vi "Configure Marker.vi"(0 "VISA resource name":refnum<visa-resource-name>, 1 "Marker X Position (1E3)":dbl=1000.0 format="%^#_9g", 2 "Enable Coupling (Disable)":bool, 3 "Enable Reference Mode (Disable)":bool, 5 "Measurement Type (6: Phase Noise)":u16(ring)=6 items=["AM Noise"=1, "Baseband Noise"=2, "Freq/Power"=3, "Spectrum"=4, "Transient"=5, "Phase Noise"=6, "User"=7], 7 "Select Trace (1: 1)":u16(ring)=1 items=["1"=1, "2"=2, "3"=3, "4"=4, "5"=5, "6"=6, "7"=7, "8"=8], 9 "Select Marker (1: 1)":u16(ring)=1 items=["1"=1, "2"=2, "3"=3, "4"=4, "5"=5, "6"=6, "7"=7, "8"=8, "9"=9, "10"=10], 11 "error in (no error)":errorcluster, 12 "Enable Marker (Enable)":bool=TRUE, 13 "Tracking Mode (4: Off)":T1(ring)=enum."Off") -> (4 "VISA resource name out":refnum<visa-resource-name>, 15 "error out":errorcluster)   [LabVIEW 2011, in "Agilent E5052X.lvlib"]
doc: "Configures markers to be used in measurements. Use multiple instances of this VI to configure multiple markers. \n\n<b>Note: </b>\n\nThis VI does not configure the search properties of the markers. Use the \"Configure Marker Search\" VI for that kind of functionality."
uses:
  Agilent E5052X.lvlib
panel:
  # "Marker Settings"
  # "Marker Function Settings"
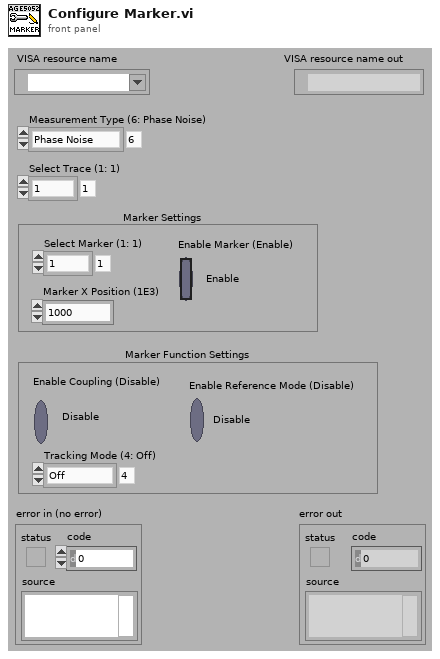
[diagram p1: front panel]
types:
  T1 = enum16{"Maximum", "Minimum", "Peak", "Target", "Off"}
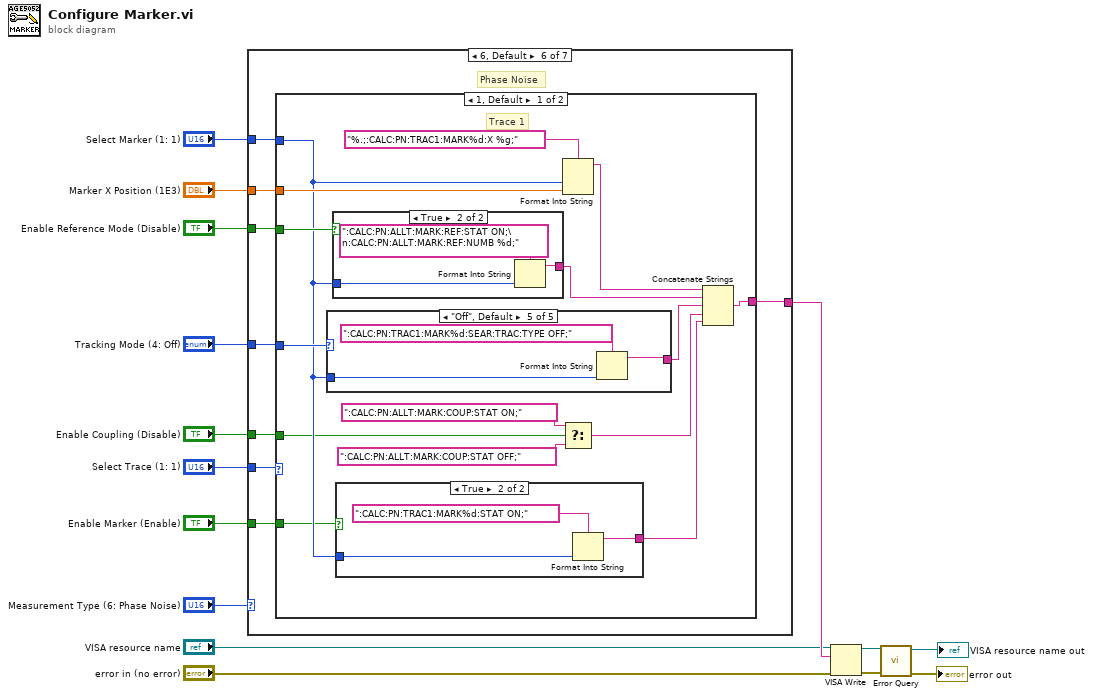
[diagram p0: block diagram]
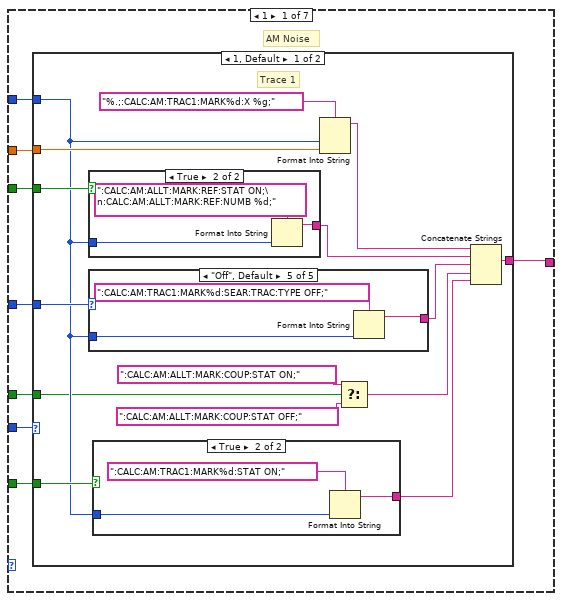
[diagram p2: hidden frame]
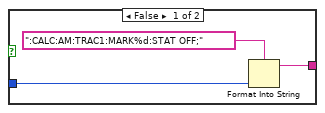
[diagram p3: hidden frame]
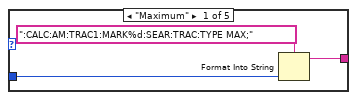
[diagram p4: hidden frame]
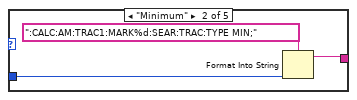
[diagram p5: hidden frame]
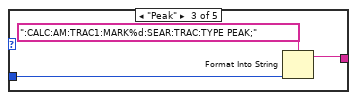
[diagram p6: hidden frame]
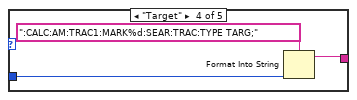
[diagram p7: hidden frame]
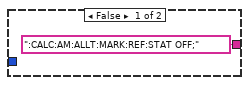
[diagram p8: hidden frame]
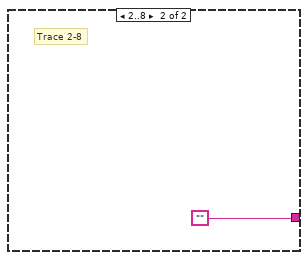
[diagram p9: hidden frame]
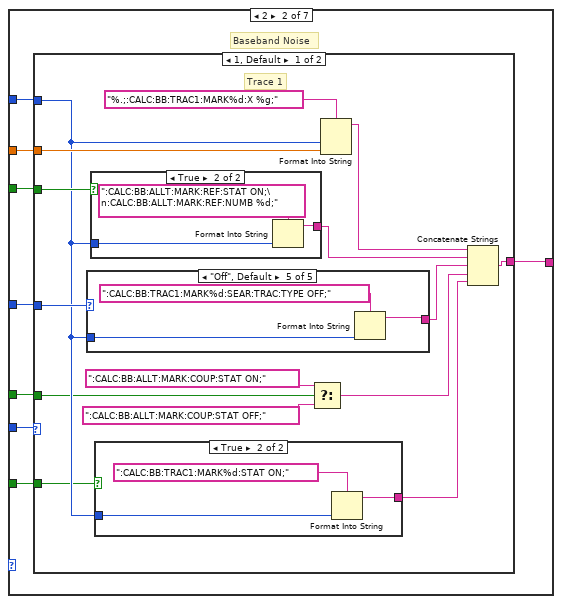
[diagram p10: hidden frame]
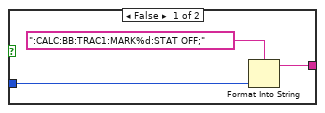
[diagram p11: hidden frame]
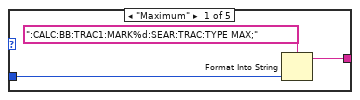
[diagram p12: hidden frame]
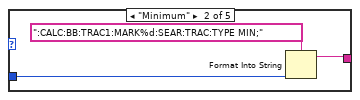
[diagram p13: hidden frame]
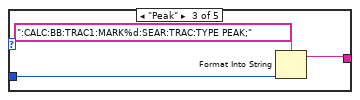
[diagram p14: hidden frame]
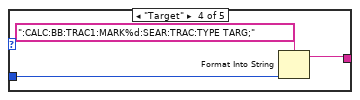
[diagram p15: hidden frame]
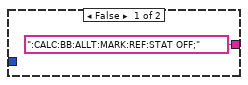
[diagram p16: hidden frame]
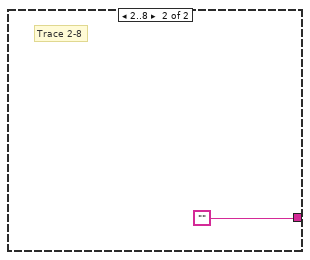
[diagram p17: hidden frame]
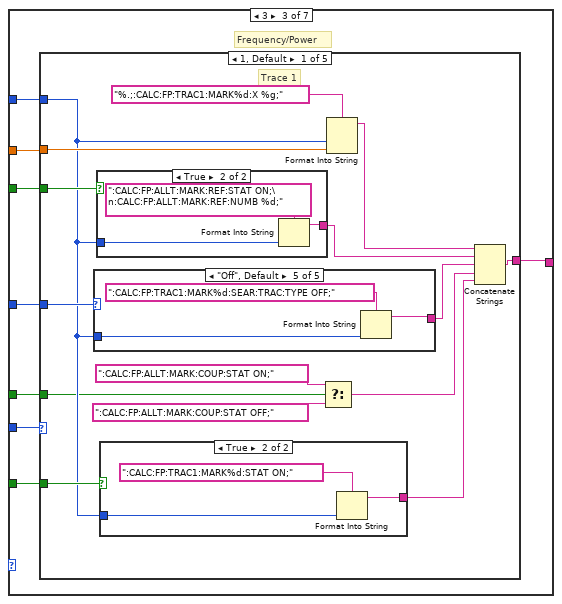
[diagram p18: hidden frame]
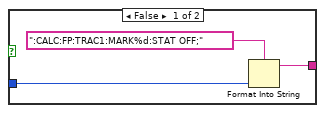
[diagram p19: hidden frame]
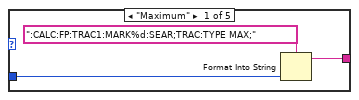
[diagram p20: hidden frame]
diagram:
  n1 = case shown="6, Default" "Measurement Type (6: Phase Noise)" {
    tunnel: "Enable Marker (Enable)" -> [w16 w65 w114 w283 w332 w501 w550]
    tunnel: "Select Trace (1: 1)" -> [w23 w67 w116 w285 w334 w503 w552]
    tunnel: "Select Marker (1: 1)" -> [w22 w72 w121 w290 w339 w508 w557]
    tunnel: "Enable Reference Mode (Disable)" -> [w21 w70 w119 w288 w337 w506 w555]
    tunnel: "Tracking Mode (4: Off)" -> [w20 w69 w118 w287 w336 w505 w554]
    tunnel: "Enable Coupling (Disable)" -> [w19 w68 w117 w286 w335 w504 w553]
    tunnel: "Marker X Position (1E3)" -> [w18 w71 w120 w289 w338 w507 w556]
    tunnel: [w17 w66 w115 w284 w333 w502 w551] -> w4
    frame 1 {
      # "AM Noise"
      n2 = case shown="1, Default" w23 {
        tunnel: w22 -> [w29 _]
        tunnel: w21 -> [w37 _]
        tunnel: w20 -> [w36 _]
        tunnel: w19 -> [w25 _]
        tunnel: w18 -> [w35 _]
        tunnel: [w31 ""] -> w17
        tunnel: w16 -> [w30 _]
        frame 1, Default {
          # "Trace 1"
          n3 = case shown="True" w37 {
            tunnel: w29 -> [_ w63]
            tunnel: [":CALC:AM:ALLT:MARK:REF:STAT OFF;" w61] -> w33
            frame False {
            }
            frame True {
              n4 = Format Into String(format string=":CALC:AM:ALLT:MARK:REF:STAT ON;\n:CALC:AM:ALLT:MARK:REF:NUMB %d;", w63) -> (resulting string=w61:string)  [unwired: 2 in, 1 out]
            }
          }
          n5 = case shown="\"Off\", Default" w36 {
            tunnel: w29 -> [w47 w49 w51 w54 w57]
            tunnel: [w45 w48 w52 w55 w58] -> w32
            frame "Maximum" {
              n6 = Format Into String(format string=":CALC:AM:TRAC1:MARK%d:SEAR:TRAC:TYPE MAX;", w47) -> (resulting string=w45:string)  [unwired: 2 in, 1 out]
            }
            frame "Minimum" {
              n7 = Format Into String(format string=":CALC:AM:TRAC1:MARK%d:SEAR:TRAC:TYPE MIN;", w49) -> (resulting string=w48:string)  [unwired: 2 in, 1 out]
            }
            frame "Peak" {
              n8 = Format Into String(format string=":CALC:AM:TRAC1:MARK%d:SEAR:TRAC:TYPE PEAK;", w51) -> (resulting string=w52:string)  [unwired: 2 in, 1 out]
            }
            frame "Target" {
              n9 = Format Into String(format string=":CALC:AM:TRAC1:MARK%d:SEAR:TRAC:TYPE TARG;", w54) -> (resulting string=w55:string)  [unwired: 2 in, 1 out]
            }
            frame "Off", Default {
              n10 = Format Into String(format string=":CALC:AM:TRAC1:MARK%d:SEAR:TRAC:TYPE OFF;", w57) -> (resulting string=w58:string)  [unwired: 2 in, 1 out]
            }
          }
          n11 = case shown="True" w30 {
            tunnel: w29 -> [w40 w43]
            tunnel: [w39 w42] -> w28
            frame False {
              n12 = Format Into String(format string=":CALC:AM:TRAC1:MARK%d:STAT OFF;", w40) -> (resulting string=w39:string)  [unwired: 2 in, 1 out]
            }
            frame True {
              n13 = Format Into String(format string=":CALC:AM:TRAC1:MARK%d:STAT ON;", w43) -> (resulting string=w42:string)  [unwired: 2 in, 1 out]
            }
          }
          n14 = Format Into String(format string="%.;:CALC:AM:TRAC1:MARK%d:X %g;", w29, w35) -> (resulting string=w34:string)  [unwired: 2 in, 1 out]
          n15 = Select(t=":CALC:AM:ALLT:MARK:COUP:STAT ON;", s=w25, f=":CALC:AM:ALLT:MARK:COUP:STAT OFF;") -> (s? t:f=w24:string)
          n16 = Concatenate Strings(w34, w33, w32, w24, w28) -> (w31:string)
        }
        frame 2..8 {
          # "Trace 2-8"
        }
      }
    }
    frame 2 {
      # "Baseband Noise"
      n17 = case shown="1, Default" w67 {
        tunnel: w72 -> [w79 _]
        tunnel: w70 -> [w86 _]
        tunnel: w69 -> [w85 _]
        tunnel: w68 -> [w74 _]
        tunnel: w71 -> [w84 _]
        tunnel: [w80 ""] -> w66
        tunnel: w65 -> [w78 _]
        frame 1, Default {
          # "Trace 1"
          n18 = case shown="\"Off\", Default" w85 {
            tunnel: w79 -> [w96 w98 w100 w103 w106]
            tunnel: [w94 w97 w101 w104 w107] -> w81
            frame "Maximum" {
              n19 = Format Into String(format string=":CALC:BB:TRAC1:MARK%d:SEAR:TRAC:TYPE MAX;", w96) -> (resulting string=w94:string)  [unwired: 2 in, 1 out]
            }
            frame "Minimum" {
              n20 = Format Into String(format string=":CALC:BB:TRAC1:MARK%d:SEAR:TRAC:TYPE MIN;", w98) -> (resulting string=w97:string)  [unwired: 2 in, 1 out]
            }
            frame "Peak" {
              n21 = Format Into String(format string=":CALC:BB:TRAC1:MARK%d:SEAR:TRAC:TYPE PEAK;", w100) -> (resulting string=w101:string)  [unwired: 2 in, 1 out]
            }
            frame "Target" {
              n22 = Format Into String(format string=":CALC:BB:TRAC1:MARK%d:SEAR:TRAC:TYPE TARG;", w103) -> (resulting string=w104:string)  [unwired: 2 in, 1 out]
            }
            frame "Off", Default {
              n23 = Format Into String(format string=":CALC:BB:TRAC1:MARK%d:SEAR:TRAC:TYPE OFF;", w106) -> (resulting string=w107:string)  [unwired: 2 in, 1 out]
            }
          }
          n24 = case shown="True" w86 {
            tunnel: w79 -> [_ w112]
            tunnel: [":CALC:BB:ALLT:MARK:REF:STAT OFF;" w110] -> w82
            frame False {
            }
            frame True {
              n25 = Format Into String(format string=":CALC:BB:ALLT:MARK:REF:STAT ON;\n:CALC:BB:ALLT:MARK:REF:NUMB %d;", w112) -> (resulting string=w110:string)  [unwired: 2 in, 1 out]
            }
          }
          n26 = case shown="True" w78 {
            tunnel: w79 -> [w89 w92]
            tunnel: [w88 w91] -> w77
            frame False {
              n27 = Format Into String(format string=":CALC:BB:TRAC1:MARK%d:STAT OFF;", w89) -> (resulting string=w88:string)  [unwired: 2 in, 1 out]
            }
            frame True {
              n28 = Format Into String(format string=":CALC:BB:TRAC1:MARK%d:STAT ON;", w92) -> (resulting string=w91:string)  [unwired: 2 in, 1 out]
            }
          }
          n29 = Select(t=":CALC:BB:ALLT:MARK:COUP:STAT ON;", s=w74, f=":CALC:BB:ALLT:MARK:COUP:STAT OFF;") -> (s? t:f=w73:string)
          n30 = Format Into String(format string="%.;:CALC:BB:TRAC1:MARK%d:X %g;", w79, w84) -> (resulting string=w83:string)  [unwired: 2 in, 1 out]
          n31 = Concatenate Strings(w83, w82, w81, w73, w77) -> (w80:string)
        }
        frame 2..8 {
          # "Trace 2-8"
        }
      }
    }
    frame 3 {
      # "Frequency/Power"
      n32 = case shown="1, Default" w116 {
        tunnel: w121 -> [w127 w168 w207 w248 _]
        tunnel: w119 -> [w135 w171 w211 w251 _]
        tunnel: w118 -> [w134 w170 w210 w250 _]
        tunnel: w117 -> [w123 w163 w203 w243 _]
        tunnel: w120 -> [w133 w172 w212 w252 _]
        tunnel: [w129 w169 w209 w249 ""] -> w115
        tunnel: w114 -> [w128 w167 w208 w247 _]
        frame 1, Default {
          # "Trace 1"
          n33 = case shown="\"Off\", Default" w134 {
            tunnel: w127 -> [w145 w147 w149 w152 w155]
            tunnel: [w143 w146 w150 w153 w156] -> w130
            frame "Maximum" {
              n34 = Format Into String(format string=":CALC:FP:TRAC1:MARK%d:SEAR;TRAC:TYPE MAX;", w145) -> (resulting string=w143:string)  [unwired: 2 in, 1 out]
            }
            frame "Minimum" {
              n35 = Format Into String(format string=":CALC:FP:TRAC1:MARK%d:SEAR;TRAC:TYPE MIN;", w147) -> (resulting string=w146:string)  [unwired: 2 in, 1 out]
            }
            frame "Peak" {
              n36 = Format Into String(format string=":CALC:FP:TRAC1:MARK%d:SEAR;TRAC:TYPE PEAK;", w149) -> (resulting string=w150:string)  [unwired: 2 in, 1 out]
            }
            frame "Target" {
              n37 = Format Into String(format string=":CALC:FP:TRAC1:MARK%d:SEAR;TRAC:TYPE TARG;", w152) -> (resulting string=w153:string)  [unwired: 2 in, 1 out]
            }
            frame "Off", Default {
              n38 = Format Into String(format string=":CALC:FP:TRAC1:MARK%d:SEAR:TRAC:TYPE OFF;", w155) -> (resulting string=w156:string)  [unwired: 2 in, 1 out]
            }
          }
          n39 = case shown="True" w135 {
            tunnel: w127 -> [_ w161]
            tunnel: [":CALC:FP:ALLT:MARK:REF:STAT OFF;" w159] -> w131
            frame False {
            }
            frame True {
              n40 = Format Into String(format string=":CALC:FP:ALLT:MARK:REF:STAT ON;\n:CALC:FP:ALLT:MARK:REF:NUMB %d;", w161) -> (resulting string=w159:string)  [unwired: 2 in, 1 out]
            }
          }
          n41 = case shown="True" w128 {
            tunnel: w127 -> [w138 w141]
            tunnel: [w137 w140] -> w126
            frame False {
              n42 = Format Into String(format string=":CALC:FP:TRAC1:MARK%d:STAT OFF;", w138) -> (resulting string=w137:string)  [unwired: 2 in, 1 out]
            }
            frame True {
              n43 = Format Into String(format string=":CALC:FP:TRAC1:MARK%d:STAT ON;", w141) -> (resulting string=w140:string)  [unwired: 2 in, 1 out]
            }
          }
          n44 = Select(t=":CALC:FP:ALLT:MARK:COUP:STAT ON;", s=w123, f=":CALC:FP:ALLT:MARK:COUP:STAT OFF;") -> (s? t:f=w122:string)
          n45 = Format Into String(format string="%.;:CALC:FP:TRAC1:MARK%d:X %g;", w127, w133) -> (resulting string=w132:string)  [unwired: 2 in, 1 out]
          n46 = Concatenate Strings(w132, w131, w130, w122, w126) -> (w129:string)
        }
        frame 2 {
          # "Trace 2"
          n47 = case shown="\"Off\", Default" w170 {
            tunnel: w168 -> [w185 w187 w189 w192 w195]
            tunnel: [w183 w186 w190 w193 w196] -> w173
            frame "Maximum" {
              n48 = Format Into String(format string=":CALC:FP:TRAC2:MARK%d:SEAR:TRAC:TYPE MAX;", w185) -> (resulting string=w183:string)  [unwired: 2 in, 1 out]
            }
            frame "Minimum" {
              n49 = Format Into String(format string=":CALC:FP:TRAC2:MARK%d:SEAR:TRAC:TYPE MIN;", w187) -> (resulting string=w186:string)  [unwired: 2 in, 1 out]
            }
            frame "Peak" {
              n50 = Format Into String(format string=":CALC:FP:TRAC2:MARK%d:SEAR:TRAC:TYPE PEAK;", w189) -> (resulting string=w190:string)  [unwired: 2 in, 1 out]
            }
            frame "Target" {
              n51 = Format Into String(format string=":CALC:FP:TRAC2:MARK%d:SEAR:TRAC:TYPE TARG;", w192) -> (resulting string=w193:string)  [unwired: 2 in, 1 out]
            }
            frame "Off", Default {
              n52 = Format Into String(format string=":CALC:FP:TRAC2:MARK%d:SEAR:TRAC:TYPE OFF;", w195) -> (resulting string=w196:string)  [unwired: 2 in, 1 out]
            }
          }
          n53 = case shown="True" w171 {
            tunnel: w168 -> [_ w201]
            tunnel: [":CALC:FP:ALLT:MARK:REF:STAT OFF;" w199] -> w174
            frame False {
            }
            frame True {
              n54 = Format Into String(format string=":CALC:FP:ALLT:MARK:REF:STAT ON;\n:CALC:FP:ALLT:MARK:REF:NUMB %d;", w201) -> (resulting string=w199:string)  [unwired: 2 in, 1 out]
            }
          }
          n55 = case shown="True" w167 {
            tunnel: w168 -> [w178 w181]
            tunnel: [w177 w180] -> w166
            frame False {
              n56 = Format Into String(format string=":CALC:FP:TRAC2:MARK%d:STAT OFF;", w178) -> (resulting string=w177:string)  [unwired: 2 in, 1 out]
            }
            frame True {
              n57 = Format Into String(format string=":CALC:FP:TRAC2:MARK%d:STAT ON;", w181) -> (resulting string=w180:string)  [unwired: 2 in, 1 out]
            }
          }
          n58 = Select(t=":CALC:FP:ALLT:MARK:COUP:STAT ON;", s=w163, f=":CALC:FP:ALLT:MARK:COUP:STAT OFF;") -> (s? t:f=w162:string)
          n59 = Format Into String(format string="%.;:CALC:FP:TRAC2:MARK%d:X %g;", w168, w172) -> (resulting string=w175:string)  [unwired: 2 in, 1 out]
          n60 = Concatenate Strings(w175, w174, w173, w162, w166) -> (w169:string)
        }
        frame 3 {
          # "Trace 3"
          n61 = case shown="\"Off\", Default" w210 {
            tunnel: w207 -> [w225 w227 w229 w232 w235]
            tunnel: [w223 w226 w230 w233 w236] -> w213
            frame "Maximum" {
              n62 = Format Into String(format string=":CALC:FP:TRAC3:MARK%d:SEAR:TRAC:TYPE MAX;", w225) -> (resulting string=w223:string)  [unwired: 2 in, 1 out]
            }
            frame "Minimum" {
              n63 = Format Into String(format string=":CALC:FP:TRAC3:MARK%d:SEAR:TRAC:TYPE MIN;", w227) -> (resulting string=w226:string)  [unwired: 2 in, 1 out]
            }
            frame "Peak" {
              n64 = Format Into String(format string=":CALC:FP:TRAC3:MARK%d:SEAR:TRAC:TYPE PEAK;", w229) -> (resulting string=w230:string)  [unwired: 2 in, 1 out]
            }
            frame "Target" {
              n65 = Format Into String(format string=":CALC:FP:TRAC3:MARK%d:SEAR:TRAC:TYPE TARG;", w232) -> (resulting string=w233:string)  [unwired: 2 in, 1 out]
            }
            frame "Off", Default {
              n66 = Format Into String(format string=":CALC:FP:TRAC3:MARK%d:SEAR:TRAC:TYPE OFF;", w235) -> (resulting string=w236:string)  [unwired: 2 in, 1 out]
            }
          }
          n67 = case shown="True" w211 {
            tunnel: w207 -> [_ w241]
            tunnel: [":CALC:FP:ALLT:MARK:REF:STAT OFF;" w239] -> w214
            frame False {
            }
            frame True {
              n68 = Format Into String(format string=":CALC:FP:ALLT:MARK:REF:STAT ON;\n:CALC:FP:ALLT:MARK:REF:NUMB %d;", w241) -> (resulting string=w239:string)  [unwired: 2 in, 1 out]
            }
          }
          n69 = case shown="True" w208 {
            tunnel: w207 -> [w218 w221]
            tunnel: [w217 w220] -> w206
            frame False {
              n70 = Format Into String(format string=":CALC:FP:TRAC3:MARK%d:STAT OFF;", w218) -> (resulting string=w217:string)  [unwired: 2 in, 1 out]
            }
            frame True {
              n71 = Format Into String(format string=":CALC:FP:TRAC3:MARK%d:STAT ON;", w221) -> (resulting string=w220:string)  [unwired: 2 in, 1 out]
            }
          }
          n72 = Format Into String(format string="%.;:CALC:FP:TRAC3:MARK%d:X %g;", w207, w212) -> (resulting string=w215:string)  [unwired: 2 in, 1 out]
          n73 = Select(t=":CALC:FP:ALLT:MARK:COUP:STAT ON;", s=w203, f=":CALC:FP:ALLT:MARK:COUP:STAT OFF;") -> (s? t:f=w202:string)
          n74 = Concatenate Strings(w215, w214, w213, w202, w206) -> (w209:string)
        }
        frame 4 {
          # "Trace 4"
          n75 = case shown="\"Off\", Default" w250 {
            tunnel: w248 -> [w265 w267 w269 w272 w275]
            tunnel: [w263 w266 w270 w273 w276] -> w253
            frame "Maximum" {
              n76 = Format Into String(format string=":CALC:FP:TRAC4:MARK%d:SEAR:TRAC:TYPE MAX;", w265) -> (resulting string=w263:string)  [unwired: 2 in, 1 out]
            }
            frame "Minimum" {
              n77 = Format Into String(format string=":CALC:FP:TRAC4:MARK%d:SEAR:TRAC:TYPE MIN;", w267) -> (resulting string=w266:string)  [unwired: 2 in, 1 out]
            }
            frame "Peak" {
              n78 = Format Into String(format string=":CALC:FP:TRAC4:MARK%d:SEAR:TRAC:TYPE PEAK;", w269) -> (resulting string=w270:string)  [unwired: 2 in, 1 out]
            }
            frame "Target" {
              n79 = Format Into String(format string=":CALC:FP:TRAC4:MARK%d:SEAR:TRAC:TYPE TARG;", w272) -> (resulting string=w273:string)  [unwired: 2 in, 1 out]
            }
            frame "Off", Default {
              n80 = Format Into String(format string=":CALC:FP:TRAC4:MARK%d:SEAR:TRAC:TYPE OFF;", w275) -> (resulting string=w276:string)  [unwired: 2 in, 1 out]
            }
          }
          n81 = case shown="True" w251 {
            tunnel: w248 -> [_ w281]
            tunnel: [":CALC:FP:ALLT:MARK:REF:STAT OFF;" w279] -> w254
            frame False {
            }
            frame True {
              n82 = Format Into String(format string=":CALC:FP:ALLT:MARK:REF:STAT ON;\n:CALC:FP:ALLT:MARK:REF:NUMB %d;", w281) -> (resulting string=w279:string)  [unwired: 2 in, 1 out]
            }
          }
          n83 = case shown="True" w247 {
            tunnel: w248 -> [w258 w261]
            tunnel: [w257 w260] -> w246
            frame False {
              n84 = Format Into String(format string=":CALC:FP:TRAC4:MARK%d:STAT OFF;", w258) -> (resulting string=w257:string)  [unwired: 2 in, 1 out]
            }
            frame True {
              n85 = Format Into String(format string=":CALC:FP:TRAC4:MARK%d:STAT ON;", w261) -> (resulting string=w260:string)  [unwired: 2 in, 1 out]
            }
          }
          n86 = Format Into String(format string="%.;:CALC:FP:TRAC4:MARK%d:X %g;", w248, w252) -> (resulting string=w255:string)  [unwired: 2 in, 1 out]
          n87 = Select(t=":CALC:FP:ALLT:MARK:COUP:STAT ON;", s=w243, f=":CALC:FP:ALLT:MARK:COUP:STAT OFF;") -> (s? t:f=w242:string)
          n88 = Concatenate Strings(w255, w254, w253, w242, w246) -> (w249:string)
        }
        frame 5..8 {
          # "Trace 5-8"
        }
      }
    }
    frame 4 {
      # "Spectrum"
      n89 = case shown="1, Default" w285 {
        tunnel: w290 -> [w295 _]
        tunnel: w288 -> [w304 _]
        tunnel: w287 -> [w303 _]
        tunnel: w286 -> [w292 _]
        tunnel: w289 -> [w302 _]
        tunnel: [w298 ""] -> w284
        tunnel: w283 -> [w297 _]
        frame 1, Default {
          # "Trace 1"
          n90 = case shown="\"Off\", Default" w303 {
            tunnel: w295 -> [w314 w316 w318 w321 w324]
            tunnel: [w312 w315 w319 w322 w325] -> w299
            frame "Maximum" {
              n91 = Format Into String(format string=":CALC:SP:TRAC1:MARK%d:SEAR:TRAC:TYPE MAX;", w314) -> (resulting string=w312:string)  [unwired: 2 in, 1 out]
            }
            frame "Minimum" {
              n92 = Format Into String(format string=":CALC:SP:TRAC1:MARK%d:SEAR:TRAC:TYPE MIN;", w316) -> (resulting string=w315:string)  [unwired: 2 in, 1 out]
            }
            frame "Peak" {
              n93 = Format Into String(format string=":CALC:SP:TRAC1:MARK%d:SEAR:TRAC:TYPE PEAK;", w318) -> (resulting string=w319:string)  [unwired: 2 in, 1 out]
            }
            frame "Target" {
              n94 = Format Into String(format string=":CALC:SP:TRAC1:MARK%d:SEAR:TRAC:TYPE TARG;", w321) -> (resulting string=w322:string)  [unwired: 2 in, 1 out]
            }
            frame "Off", Default {
              n95 = Format Into String(format string=":CALC:SP:TRAC1:MARK%d:SEAR:TRAC:TYPE OFF;", w324) -> (resulting string=w325:string)  [unwired: 2 in, 1 out]
            }
          }
          n96 = case shown="True" w304 {
            tunnel: w295 -> [_ w330]
            tunnel: [":CALC:SP:ALLT:MARK:REF:STAT OFF;" w328] -> w300
            frame False {
            }
            frame True {
              n97 = Format Into String(format string=":CALC:SP:ALLT:MARK:REF:STAT ON;\n:CALC:SP:ALLT:MARK:REF:NUMB %d;", w330) -> (resulting string=w328:string)  [unwired: 2 in, 1 out]
            }
          }
          n98 = case shown="True" w297 {
            tunnel: w295 -> [w307 w310]
            tunnel: [w306 w309] -> w296
            frame False {
              n99 = Format Into String(format string=":CALC:SP:TRAC1:MARK%d:STAT OFF;", w307) -> (resulting string=w306:string)  [unwired: 2 in, 1 out]
            }
            frame True {
              n100 = Format Into String(format string=":CALC:SP:TRAC1:MARK%d:STAT ON;", w310) -> (resulting string=w309:string)  [unwired: 2 in, 1 out]
            }
          }
          n101 = Format Into String(format string="%.;:CALC:SP:TRAC1:MARK%d:X %g;", w295, w302) -> (resulting string=w301:string)  [unwired: 2 in, 1 out]
          n102 = Select(t=":CALC:SP:ALLT:MARK:COUP:STAT ON;", s=w292, f=":CALC:SP:ALLT:MARK:COUP:STAT OFF;") -> (s? t:f=w291:string)
          n103 = Concatenate Strings(w301, w300, w299, w291, w296) -> (w298:string)
        }
        frame 2..8 {
          # "Trace 2-8"
        }
      }
    }
    frame 5 {
      # "Transient"
      n104 = case shown="1, Default" w334 {
        tunnel: w339 -> [w344 w385 w425 w465 _]
        tunnel: w337 -> [w353 w389 w429 w469 _]
        tunnel: w336 -> [w352 w388 w428 w468 _]
        tunnel: w335 -> [w341 w381 w421 w461 _]
        tunnel: w338 -> [w351 w390 w430 w470 _]
        tunnel: [w347 w387 w427 w467 ""] -> w333
        tunnel: w332 -> [w345 w386 w426 w466 _]
        frame 1, Default {
          # "Trace 1"
          n105 = case shown="\"Off\", Default" w352 {
            tunnel: w344 -> [w363 w365 w367 w370 w373]
            tunnel: [w361 w364 w368 w371 w374] -> w348
            frame "Maximum" {
              n106 = Format Into String(format string=":CALC:TR:TRAC1:MARK%d:SEAR:TRAC:TYPE MAX;", w363) -> (resulting string=w361:string)  [unwired: 2 in, 1 out]
            }
            frame "Minimum" {
              n107 = Format Into String(format string=":CALC:TR:TRAC1:MARK%d:SEAR:TRAC:TYPE MIN;", w365) -> (resulting string=w364:string)  [unwired: 2 in, 1 out]
            }
            frame "Peak" {
              n108 = Format Into String(format string=":CALC:TR:TRAC1:MARK%d:SEAR:TRAC:TYPE PEAK;", w367) -> (resulting string=w368:string)  [unwired: 2 in, 1 out]
            }
            frame "Target" {
              n109 = Format Into String(format string=":CALC:TR:TRAC1:MARK%d:SEAR:TRAC:TYPE TARG;", w370) -> (resulting string=w371:string)  [unwired: 2 in, 1 out]
            }
            frame "Off", Default {
              n110 = Format Into String(format string=":CALC:TR:TRAC1:MARK%d:SEAR:TRAC:TYPE OFF;", w373) -> (resulting string=w374:string)  [unwired: 2 in, 1 out]
            }
          }
          n111 = case shown="True" w353 {
            tunnel: w344 -> [_ w379]
            tunnel: [":CALC:TR:ALLT:MARK:REF:STAT OFF;" w377] -> w349
            frame False {
            }
            frame True {
              n112 = Format Into String(format string=":CALC:TR:ALLT:MARK:REF:STAT ON;\n:CALC:TR:ALLT:MARK:REF:NUMB %d;", w379) -> (resulting string=w377:string)  [unwired: 2 in, 1 out]
            }
          }
          n113 = case shown="True" w345 {
            tunnel: w344 -> [w356 w359]
            tunnel: [w355 w358] -> w346
            frame False {
              n114 = Format Into String(format string=":CALC:TR:TRAC1:MARK%d:STAT OFF;", w356) -> (resulting string=w355:string)  [unwired: 2 in, 1 out]
            }
            frame True {
              n115 = Format Into String(format string=":CALC:TR:TRAC1:MARK%d:STAT ON;", w359) -> (resulting string=w358:string)  [unwired: 2 in, 1 out]
            }
          }
          n116 = Format Into String(format string="%.;:CALC:TR:TRAC1:MARK%d:X %g;", w344, w351) -> (resulting string=w350:string)  [unwired: 2 in, 1 out]
          n117 = Select(t=":CALC:TR:ALLT:MARK:COUP:STAT ON;", s=w341, f=":CALC:TR:ALLT:MARK:COUP:STAT OFF;") -> (s? t:f=w340:string)
          n118 = Concatenate Strings(w350, w349, w348, w340, w346) -> (w347:string)
        }
        frame 2 {
          # "Trace 2"
          n119 = case shown="\"Off\", Default" w388 {
            tunnel: w385 -> [w403 w405 w407 w410 w413]
            tunnel: [w401 w404 w408 w411 w414] -> w391
            frame "Maximum" {
              n120 = Format Into String(format string=":CALC:TR:TRAC2:MARK%d:SEAR:TRAC:TYPE MAX;", w403) -> (resulting string=w401:string)  [unwired: 2 in, 1 out]
            }
            frame "Minimum" {
              n121 = Format Into String(format string=":CALC:TR:TRAC2:MARK%d:SEAR:TRAC:TYPE MIN;", w405) -> (resulting string=w404:string)  [unwired: 2 in, 1 out]
            }
            frame "Peak" {
              n122 = Format Into String(format string=":CALC:TR:TRAC2:MARK%d:SEAR:TRAC:TYPE PEAK;", w407) -> (resulting string=w408:string)  [unwired: 2 in, 1 out]
            }
            frame "Target" {
              n123 = Format Into String(format string=":CALC:TR:TRAC2:MARK%d:SEAR:TRAC:TYPE TARG;", w410) -> (resulting string=w411:string)  [unwired: 2 in, 1 out]
            }
            frame "Off", Default {
              n124 = Format Into String(format string=":CALC:TR:TRAC2:MARK%d:SEAR:TRAC:TYPE OFF;", w413) -> (resulting string=w414:string)  [unwired: 2 in, 1 out]
            }
          }
          n125 = case shown="True" w389 {
            tunnel: w385 -> [_ w419]
            tunnel: [":CALC:TR:ALLT:MARK:REF:STAT OFF;" w417] -> w392
            frame False {
            }
            frame True {
              n126 = Format Into String(format string=":CALC:TR:ALLT:MARK:REF:STAT ON;\n:CALC:TR:ALLT:MARK:REF:NUMB %d;", w419) -> (resulting string=w417:string)  [unwired: 2 in, 1 out]
            }
          }
          n127 = case shown="True" w386 {
            tunnel: w385 -> [w396 w399]
            tunnel: [w395 w398] -> w384
            frame False {
              n128 = Format Into String(format string=":CALC:TR:TRAC2:MARK%d:STAT OFF;", w396) -> (resulting string=w395:string)  [unwired: 2 in, 1 out]
            }
            frame True {
              n129 = Format Into String(format string=":CALC:TR:TRAC2:MARK%d:STAT ON;", w399) -> (resulting string=w398:string)  [unwired: 2 in, 1 out]
            }
          }
          n130 = Select(t=":CALC:TR:ALLT:MARK:COUP:STAT ON;", s=w381, f=":CALC:TR:ALLT:MARK:COUP:STAT OFF;") -> (s? t:f=w380:string)
          n131 = Format Into String(format string="%.;:CALC:TR:TRAC2:MARK%d:X %g;", w385, w390) -> (resulting string=w393:string)  [unwired: 2 in, 1 out]
          n132 = Concatenate Strings(w393, w392, w391, w380, w384) -> (w387:string)
        }
        frame 3 {
          # "Trace 3"
          n133 = case shown="\"Off\", Default" w428 {
            tunnel: w425 -> [w443 w445 w447 w450 w453]
            tunnel: [w441 w444 w448 w451 w454] -> w431
            frame "Maximum" {
              n134 = Format Into String(format string=":CALC:TR:TRAC3:MARK%d:SEAR:TRAC:TYPE MAX;", w443) -> (resulting string=w441:string)  [unwired: 2 in, 1 out]
            }
            frame "Minimum" {
              n135 = Format Into String(format string=":CALC:TR:TRAC3:MARK%d:SEAR:TRAC:TYPE MIN;", w445) -> (resulting string=w444:string)  [unwired: 2 in, 1 out]
            }
            frame "Peak" {
              n136 = Format Into String(format string=":CALC:TR:TRAC3:MARK%d:SEAR:TRAC:TYPE PEAK;", w447) -> (resulting string=w448:string)  [unwired: 2 in, 1 out]
            }
            frame "Target" {
              n137 = Format Into String(format string=":CALC:TR:TRAC3:MARK%d:SEAR:TRAC:TYPE TARG;", w450) -> (resulting string=w451:string)  [unwired: 2 in, 1 out]
            }
            frame "Off", Default {
              n138 = Format Into String(format string=":CALC:TR:TRAC3:MARK%d:SEAR:TRAC:TYPE OFF;", w453) -> (resulting string=w454:string)  [unwired: 2 in, 1 out]
            }
          }
          n139 = case shown="True" w429 {
            tunnel: w425 -> [_ w459]
            tunnel: [":CALC:TR:ALLT:MARK:REF:STAT OFF;" w457] -> w432
            frame False {
            }
            frame True {
              n140 = Format Into String(format string=":CALC:TR:ALLT:MARK:REF:STAT ON;\n:CALC:TR:ALLT:MARK:REF:NUMB %d;", w459) -> (resulting string=w457:string)  [unwired: 2 in, 1 out]
            }
          }
          n141 = case shown="True" w426 {
            tunnel: w425 -> [w436 w439]
            tunnel: [w435 w438] -> w424
            frame False {
              n142 = Format Into String(format string=":CALC:TR:TRAC3:MARK%d:STAT OFF;", w436) -> (resulting string=w435:string)  [unwired: 2 in, 1 out]
            }
            frame True {
              n143 = Format Into String(format string=":CALC:TR:TRAC3:MARK%d:STAT ON;", w439) -> (resulting string=w438:string)  [unwired: 2 in, 1 out]
            }
          }
          n144 = Format Into String(format string="%.;:CALC:TR:TRAC3:MARK%d:X %g;", w425, w430) -> (resulting string=w433:string)  [unwired: 2 in, 1 out]
          n145 = Select(t=":CALC:TR:ALLT:MARK:COUP:STAT ON;", s=w421, f=":CALC:TR:ALLT:MARK:COUP:STAT OFF;") -> (s? t:f=w420:string)
          n146 = Concatenate Strings(w433, w432, w431, w420, w424) -> (w427:string)
        }
        frame 4 {
          # "Trace 4"
          n147 = case shown="\"Off\", Default" w468 {
            tunnel: w465 -> [w483 w485 w487 w490 w493]
            tunnel: [w481 w484 w488 w491 w494] -> w471
            frame "Maximum" {
              n148 = Format Into String(format string=":CALC:TR:TRAC4:MARK%d:SEAR:TRAC:TYPE MAX;", w483) -> (resulting string=w481:string)  [unwired: 2 in, 1 out]
            }
            frame "Minimum" {
              n149 = Format Into String(format string=":CALC:TR:TRAC4:MARK%d:SEAR:TRAC:TYPE MIN;", w485) -> (resulting string=w484:string)  [unwired: 2 in, 1 out]
            }
            frame "Peak" {
              n150 = Format Into String(format string=":CALC:TR:TRAC4:MARK%d:SEAR:TRAC:TYPE PEAK;", w487) -> (resulting string=w488:string)  [unwired: 2 in, 1 out]
            }
            frame "Target" {
              n151 = Format Into String(format string=":CALC:TR:TRAC4:MARK%d:SEAR:TRAC:TYPE TARG;", w490) -> (resulting string=w491:string)  [unwired: 2 in, 1 out]
            }
            frame "Off", Default {
              n152 = Format Into String(format string=":CALC:TR:TRAC4:MARK%d:SEAR:TRAC:TYPE OFF;", w493) -> (resulting string=w494:string)  [unwired: 2 in, 1 out]
            }
          }
          n153 = case shown="True" w469 {
            tunnel: w465 -> [_ w499]
            tunnel: [":CALC:TR:ALLT:MARK:REF:STAT OFF;" w497] -> w472
            frame False {
            }
            frame True {
              n154 = Format Into String(format string=":CALC:TR:ALLT:MARK:REF:STAT ON;\n:CALC:TR:ALLT:MARK:REF:NUMB %d;", w499) -> (resulting string=w497:string)  [unwired: 2 in, 1 out]
            }
          }
          n155 = case shown="True" w466 {
            tunnel: w465 -> [w476 w479]
            tunnel: [w475 w478] -> w464
            frame False {
              n156 = Format Into String(format string=":CALC:TR:TRAC4:MARK%d:STAT OFF;", w476) -> (resulting string=w475:string)  [unwired: 2 in, 1 out]
            }
            frame True {
              n157 = Format Into String(format string=":CALC:TR:TRAC4:MARK%d:STAT ON;", w479) -> (resulting string=w478:string)  [unwired: 2 in, 1 out]
            }
          }
          n158 = Format Into String(format string="%.;:CALC:TR:TRAC4:MARK%d:X %g;", w465, w470) -> (resulting string=w473:string)  [unwired: 2 in, 1 out]
          n159 = Select(t=":CALC:TR:ALLT:MARK:COUP:STAT ON;", s=w461, f=":CALC:TR:ALLT:MARK:COUP:STAT OFF;") -> (s? t:f=w460:string)
          n160 = Concatenate Strings(w473, w472, w471, w460, w464) -> (w467:string)
        }
        frame 5..8 {
          # "Trace 5-8"
        }
      }
    }
    frame 6, Default {
      # "Phase Noise"
      n161 = case shown="1, Default" w503 {
        tunnel: w508 -> [w515 _]
        tunnel: w506 -> [w522 _]
        tunnel: w505 -> [w521 _]
        tunnel: w504 -> [w510 _]
        tunnel: w507 -> [w520 _]
        tunnel: [w516 ""] -> w502
        tunnel: w501 -> [w513 _]
        frame 1, Default {
          # "Trace 1"
          n162 = case shown="\"Off\", Default" w521 {
            tunnel: w515 -> [w532 w534 w536 w539 w542]
            tunnel: [w530 w533 w537 w540 w543] -> w517
            frame "Maximum" {
              n163 = Format Into String(format string=":CALC:PN:TRAC1:MARK%d:SEAR:TRAC:TYPE MAX;", w532) -> (resulting string=w530:string)  [unwired: 2 in, 1 out]
            }
            frame "Minimum" {
              n164 = Format Into String(format string=":CALC:PN:TRAC1:MARK%d:SEAR:TRAC:TYPE MIN;", w534) -> (resulting string=w533:string)  [unwired: 2 in, 1 out]
            }
            frame "Peak" {
              n165 = Format Into String(format string=":CALC:PN:TRAC1:MARK%d:SEAR:TRAC:TYPE PEAK;", w536) -> (resulting string=w537:string)  [unwired: 2 in, 1 out]
            }
            frame "Target" {
              n166 = Format Into String(format string=":CALC:PN:TRAC1:MARK%d:SEAR:TRAC:TYPE TARG;", w539) -> (resulting string=w540:string)  [unwired: 2 in, 1 out]
            }
            frame "Off", Default {
              n167 = Format Into String(format string=":CALC:PN:TRAC1:MARK%d:SEAR:TRAC:TYPE OFF;", w542) -> (resulting string=w543:string)  [unwired: 2 in, 1 out]
            }
          }
          n168 = case shown="True" w522 {
            tunnel: w515 -> [_ w548]
            tunnel: [":CALC:PN:ALLT:MARK:REF:STAT OFF;" w546] -> w518
            frame False {
            }
            frame True {
              n169 = Format Into String(format string=":CALC:PN:ALLT:MARK:REF:STAT ON;\n:CALC:PN:ALLT:MARK:REF:NUMB %d;", w548) -> (resulting string=w546:string)  [unwired: 2 in, 1 out]
            }
          }
          n170 = case shown="True" w513 {
            tunnel: w515 -> [w525 w528]
            tunnel: [w524 w527] -> w514
            frame False {
              n171 = Format Into String(format string=":CALC:PN:TRAC1:MARK%d:STAT OFF;", w525) -> (resulting string=w524:string)  [unwired: 2 in, 1 out]
            }
            frame True {
              n172 = Format Into String(format string=":CALC:PN:TRAC1:MARK%d:STAT ON;", w528) -> (resulting string=w527:string)  [unwired: 2 in, 1 out]
            }
          }
          n173 = Format Into String(format string="%.;:CALC:PN:TRAC1:MARK%d:X %g;", w515, w520) -> (resulting string=w519:string)  [unwired: 2 in, 1 out]
          n174 = Select(t=":CALC:PN:ALLT:MARK:COUP:STAT ON;", s=w510, f=":CALC:PN:ALLT:MARK:COUP:STAT OFF;") -> (s? t:f=w509:string)
          n175 = Concatenate Strings(w519, w518, w517, w509, w514) -> (w516:string)
        }
        frame 2..8 {
          # "Trace 2-8"
        }
      }
    }
    frame 7 {
      # "User"
      n176 = case shown="1, Default" w552 {
        tunnel: w557 -> [w563 w604 w643 w682 w724 w763 w804 w843]
        tunnel: w555 -> [w571 w607 w647 w687 w727 w767 w807 w847]
        tunnel: w554 -> [w570 w606 w646 w686 w726 w766 w806 w846]
        tunnel: w553 -> [w559 w599 w639 w679 w719 w759 w799 w840]
        tunnel: w556 -> [w569 w608 w648 w688 w728 w768 w808 w848]
        tunnel: [w565 w605 w645 w685 w725 w765 w805 w845] -> w551
        tunnel: w550 -> [w564 w603 w644 w683 w723 w764 w803 w844]
        frame 1, Default {
          # "Trace 1"
          n177 = case shown="\"Off\", Default" w570 {
            tunnel: w563 -> [w581 w583 w585 w588 w591]
            tunnel: [w579 w582 w586 w589 w592] -> w566
            frame "Maximum" {
              n178 = Format Into String(format string=":CALC:USER:TRAC1:MARK%d:SEAR:TRAC:TYPE MAX;", w581) -> (resulting string=w579:string)  [unwired: 2 in, 1 out]
            }
            frame "Minimum" {
              n179 = Format Into String(format string=":CALC:USER:TRAC1:MARK%d:SEAR:TRAC:TYPE MIN;", w583) -> (resulting string=w582:string)  [unwired: 2 in, 1 out]
            }
            frame "Peak" {
              n180 = Format Into String(format string=":CALC:USER:TRAC1:MARK%d:SEAR:TRAC:TYPE PEAK;", w585) -> (resulting string=w586:string)  [unwired: 2 in, 1 out]
            }
            frame "Target" {
              n181 = Format Into String(format string=":CALC:USER:TRAC1:MARK%d:SEAR:TRAC:TYPE TARG;", w588) -> (resulting string=w589:string)  [unwired: 2 in, 1 out]
            }
            frame "Off", Default {
              n182 = Format Into String(format string=":CALC:USER:TRAC1:MARK%d:SEAR:TRAC:TYPE OFF;", w591) -> (resulting string=w592:string)  [unwired: 2 in, 1 out]
            }
          }
          n183 = case shown="True" w571 {
            tunnel: w563 -> [_ w597]
            tunnel: [":CALC:USER:ALLT:MARK:REF:STAT OFF;" w595] -> w567
            frame False {
            }
            frame True {
              n184 = Format Into String(format string=":CALC:USER:ALLT:MARK:REF:STAT ON;\n:CALC:USER:ALLT:MARK:REF:NUMB %d;", w597) -> (resulting string=w595:string)  [unwired: 2 in, 1 out]
            }
          }
          n185 = case shown="True" w564 {
            tunnel: w563 -> [w574 w577]
            tunnel: [w573 w576] -> w562
            frame False {
              n186 = Format Into String(format string=":CALC:USER:TRAC1:MARK%d:STAT OFF;", w574) -> (resulting string=w573:string)  [unwired: 2 in, 1 out]
            }
            frame True {
              n187 = Format Into String(format string=":CALC:USER:TRAC1:MARK%d:STAT ON;", w577) -> (resulting string=w576:string)  [unwired: 2 in, 1 out]
            }
          }
          n188 = Select(t=":CALC:USER:ALLT:MARK:COUP:STAT ON;", s=w559, f=":CALC:USER:ALLT:MARK:COUP:STAT OFF;") -> (s? t:f=w558:string)
          n189 = Format Into String(format string="%.;:CALC:USER:TRAC1:MARK%d:X %g;", w563, w569) -> (resulting string=w568:string)  [unwired: 2 in, 1 out]
          n190 = Concatenate Strings(w568, w567, w566, w558, w562) -> (w565:string)
        }
        frame 2 {
          # "Trace 2"
          n191 = case shown="\"Minimum\"" w606 {
            tunnel: w604 -> [w621 w623 w625 w628 w631]
            tunnel: [w619 w622 w626 w629 w632] -> w609
            frame "Maximum" {
              n192 = Format Into String(format string=":CALC:USER:TRAC2:MARK%d:SEAR:TRAC:TYPE MAX;", w621) -> (resulting string=w619:string)  [unwired: 2 in, 1 out]
            }
            frame "Minimum" {
              n193 = Format Into String(format string=":CALC:USER:TRAC2:MARK%d:SEAR:TRAC:TYPE MIN;", w623) -> (resulting string=w622:string)  [unwired: 2 in, 1 out]
            }
            frame "Peak" {
              n194 = Format Into String(format string=":CALC:USER:TRAC2:MARK%d:SEAR:TRAC:TYPE PEAK;", w625) -> (resulting string=w626:string)  [unwired: 2 in, 1 out]
            }
            frame "Target" {
              n195 = Format Into String(format string=":CALC:USER:TRAC2:MARK%d:SEAR:TRAC:TYPE TARG;", w628) -> (resulting string=w629:string)  [unwired: 2 in, 1 out]
            }
            frame "Off", Default {
              n196 = Format Into String(format string=":CALC:USER:TRAC2:MARK%d:SEAR:TRAC:TYPE OFF;", w631) -> (resulting string=w632:string)  [unwired: 2 in, 1 out]
            }
          }
          n197 = case shown="True" w607 {
            tunnel: w604 -> [_ w637]
            tunnel: [":CALC:USER:ALLT:MARK:REF:STAT OFF;" w635] -> w610
            frame False {
            }
            frame True {
              n198 = Format Into String(format string=":CALC:USER:ALLT:MARK:REF:STAT ON;\n:CALC:USER:ALLT:MARK:REF:NUMB %d;", w637) -> (resulting string=w635:string)  [unwired: 2 in, 1 out]
            }
          }
          n199 = case shown="True" w603 {
            tunnel: w604 -> [w614 w617]
            tunnel: [w613 w616] -> w602
            frame False {
              n200 = Format Into String(format string=":CALC:USER:TRAC2:MARK%d:STAT OFF;", w614) -> (resulting string=w613:string)  [unwired: 2 in, 1 out]
            }
            frame True {
              n201 = Format Into String(format string=":CALC:USER:TRAC2:MARK%d:STAT ON;", w617) -> (resulting string=w616:string)  [unwired: 2 in, 1 out]
            }
          }
          n202 = Select(t=":CALC:USER:ALLT:MARK:COUP:STAT ON;", s=w599, f=":CALC:USER:ALLT:MARK:COUP:STAT OFF;") -> (s? t:f=w598:string)
          n203 = Format Into String(format string="%.;:CALC:USER:TRAC2:MARK%d:X %g;", w604, w608) -> (resulting string=w611:string)  [unwired: 2 in, 1 out]
          n204 = Concatenate Strings(w611, w610, w609, w598, w602) -> (w605:string)
        }
        frame 3 {
          # "Trace 3"
          n205 = case shown="\"Off\", Default" w646 {
            tunnel: w643 -> [w661 w663 w665 w668 w671]
            tunnel: [w659 w662 w666 w669 w672] -> w649
            frame "Maximum" {
              n206 = Format Into String(format string=":CALC:USER:TRAC3:MARK%d:SEAR:TRAC:TYPE MAX;", w661) -> (resulting string=w659:string)  [unwired: 2 in, 1 out]
            }
            frame "Minimum" {
              n207 = Format Into String(format string=":CALC:USER:TRAC3:MARK%d:SEAR:TRAC:TYPE MIN;", w663) -> (resulting string=w662:string)  [unwired: 2 in, 1 out]
            }
            frame "Peak" {
              n208 = Format Into String(format string=":CALC:USER:TRAC3:MARK%d:SEAR:TRAC:TYPE PEAK;", w665) -> (resulting string=w666:string)  [unwired: 2 in, 1 out]
            }
            frame "Target" {
              n209 = Format Into String(format string=":CALC:USER:TRAC3:MARK%d:SEAR:TRAC:TYPE TARG;", w668) -> (resulting string=w669:string)  [unwired: 2 in, 1 out]
            }
            frame "Off", Default {
              n210 = Format Into String(format string=":CALC:USER:TRAC3:MARK%d:SEAR:TRAC:TYPE OFF;", w671) -> (resulting string=w672:string)  [unwired: 2 in, 1 out]
            }
          }
          n211 = case shown="True" w647 {
            tunnel: w643 -> [_ w677]
            tunnel: [":CALC:USER:ALLT:MARK:REF:STAT OFF;" w675] -> w650
            frame False {
            }
            frame True {
              n212 = Format Into String(format string=":CALC:USER:ALLT:MARK:REF:STAT ON;\n:CALC:USER:ALLT:MARK:REF:NUMB %d;", w677) -> (resulting string=w675:string)  [unwired: 2 in, 1 out]
            }
          }
          n213 = case shown="True" w644 {
            tunnel: w643 -> [w654 w657]
            tunnel: [w653 w656] -> w642
            frame False {
              n214 = Format Into String(format string=":CALC:USER:TRAC3:MARK%d:STAT OFF;", w654) -> (resulting string=w653:string)  [unwired: 2 in, 1 out]
            }
            frame True {
              n215 = Format Into String(format string=":CALC:USER:TRAC3:MARK%d:STAT ON;", w657) -> (resulting string=w656:string)  [unwired: 2 in, 1 out]
            }
          }
          n216 = Format Into String(format string="%.;:CALC:USER:TRAC3:MARK%d:X %g;", w643, w648) -> (resulting string=w651:string)  [unwired: 2 in, 1 out]
          n217 = Select(t=":CALC:USER:ALLT:MARK:COUP:STAT ON;", s=w639, f=":CALC:USER:ALLT:MARK:COUP:STAT OFF;") -> (s? t:f=w638:string)
          n218 = Concatenate Strings(w651, w650, w649, w638, w642) -> (w645:string)
        }
        frame 4 {
          # "Trace 4"
          n219 = case shown="\"Off\", Default" w686 {
            tunnel: w682 -> [w701 w703 w705 w708 w711]
            tunnel: [w699 w702 w706 w709 w712] -> w689
            frame "Maximum" {
              n220 = Format Into String(format string=":CALC:USER:TRAC4:MARK%d:SEAR:TRAC:TYPE MAX;", w701) -> (resulting string=w699:string)  [unwired: 2 in, 1 out]
            }
            frame "Minimum" {
              n221 = Format Into String(format string=":CALC:USER:TRAC4:MARK%d:SEAR:TRAC:TYPE MIN;", w703) -> (resulting string=w702:string)  [unwired: 2 in, 1 out]
            }
            frame "Peak" {
              n222 = Format Into String(format string=":CALC:USER:TRAC4:MARK%d:SEAR:TRAC:TYPE PEAK;", w705) -> (resulting string=w706:string)  [unwired: 2 in, 1 out]
            }
            frame "Target" {
              n223 = Format Into String(format string=":CALC:USER:TRAC4:MARK%d:SEAR:TRAC:TYPE TARG;", w708) -> (resulting string=w709:string)  [unwired: 2 in, 1 out]
            }
            frame "Off", Default {
              n224 = Format Into String(format string=":CALC:USER:TRAC4:MARK%d:SEAR:TRAC:TYPE OFF;", w711) -> (resulting string=w712:string)  [unwired: 2 in, 1 out]
            }
          }
          n225 = case shown="True" w687 {
            tunnel: w682 -> [_ w717]
            tunnel: [":CALC:USER:ALLT:MARK:REF:STAT OFF;" w715] -> w690
            frame False {
            }
            frame True {
              n226 = Format Into String(format string=":CALC:USER:ALLT:MARK:REF:STAT ON;\n:CALC:USER:ALLT:MARK:REF:NUMB %d;", w717) -> (resulting string=w715:string)  [unwired: 2 in, 1 out]
            }
          }
          n227 = case shown="True" w683 {
            tunnel: w682 -> [w694 w697]
            tunnel: [w693 w696] -> w684
            frame False {
              n228 = Format Into String(format string=":CALC:USER:TRAC4:MARK%d:STAT OFF;", w694) -> (resulting string=w693:string)  [unwired: 2 in, 1 out]
            }
            frame True {
              n229 = Format Into String(format string=":CALC:USER:TRAC4:MARK%d:STAT ON;", w697) -> (resulting string=w696:string)  [unwired: 2 in, 1 out]
            }
          }
          n230 = Format Into String(format string="%.;:CALC:USER:TRAC4:MARK%d:X %g;", w682, w688) -> (resulting string=w691:string)  [unwired: 2 in, 1 out]
          n231 = Select(t=":CALC:USER:ALLT:MARK:COUP:STAT ON;", s=w679, f=":CALC:USER:ALLT:MARK:COUP:STAT OFF;") -> (s? t:f=w678:string)
          n232 = Concatenate Strings(w691, w690, w689, w678, w684) -> (w685:string)
        }
        frame 5 {
          # "Trace 5"
          n233 = case shown="\"Off\", Default" w726 {
            tunnel: w724 -> [w741 w743 w745 w748 w751]
            tunnel: [w739 w742 w746 w749 w752] -> w729
            frame "Maximum" {
              n234 = Format Into String(format string=":CALC:USER:TRAC5:MARK%d:SEAR:TRAC:TYPE MAX;", w741) -> (resulting string=w739:string)  [unwired: 2 in, 1 out]
            }
            frame "Minimum" {
              n235 = Format Into String(format string=":CALC:USER:TRAC5:MARK%d:SEAR:TRAC:TYPE MIN;", w743) -> (resulting string=w742:string)  [unwired: 2 in, 1 out]
            }
            frame "Peak" {
              n236 = Format Into String(format string=":CALC:USER:TRAC5:MARK%d:SEAR:TRAC:TYPE PEAK;", w745) -> (resulting string=w746:string)  [unwired: 2 in, 1 out]
            }
            frame "Target" {
              n237 = Format Into String(format string=":CALC:USER:TRAC5:MARK%d:SEAR:TRAC:TYPE TARG;", w748) -> (resulting string=w749:string)  [unwired: 2 in, 1 out]
            }
            frame "Off", Default {
              n238 = Format Into String(format string=":CALC:USER:TRAC5:MARK%d:SEAR:TRAC:TYPE OFF;", w751) -> (resulting string=w752:string)  [unwired: 2 in, 1 out]
            }
          }
          n239 = case shown="True" w727 {
            tunnel: w724 -> [_ w757]
            tunnel: [":CALC:USER:ALLT:MARK:REF:STAT OFF;" w755] -> w730
            frame False {
            }
            frame True {
              n240 = Format Into String(format string=":CALC:USER:ALLT:MARK:REF:STAT ON;\n:CALC:USER:ALLT:MARK:REF:NUMB %d;", w757) -> (resulting string=w755:string)  [unwired: 2 in, 1 out]
            }
          }
          n241 = case shown="True" w723 {
            tunnel: w724 -> [w734 w737]
            tunnel: [w733 w736] -> w722
            frame False {
              n242 = Format Into String(format string=":CALC:USER:TRAC5:MARK%d:STAT OFF;", w734) -> (resulting string=w733:string)  [unwired: 2 in, 1 out]
            }
            frame True {
              n243 = Format Into String(format string=":CALC:USER:TRAC5:MARK%d:STAT ON;", w737) -> (resulting string=w736:string)  [unwired: 2 in, 1 out]
            }
          }
          n244 = Format Into String(format string="%.;:CALC:USER:TRAC5:MARK%d:X %g;", w724, w728) -> (resulting string=w731:string)  [unwired: 2 in, 1 out]
          n245 = Select(t=":CALC:USER:ALLT:MARK:COUP:STAT ON;", s=w719, f=":CALC:USER:ALLT:MARK:COUP:STAT OFF;") -> (s? t:f=w718:string)
          n246 = Concatenate Strings(w731, w730, w729, w718, w722) -> (w725:string)
        }
        frame 6 {
          # "Trace 6"
          n247 = case shown="\"Off\", Default" w766 {
            tunnel: w763 -> [w781 w783 w785 w788 w791]
            tunnel: [w779 w782 w786 w789 w792] -> w769
            frame "Maximum" {
              n248 = Format Into String(format string=":CALC:USER:TRAC6:MARK%d:SEAR:TRAC:TYPE MAX;", w781) -> (resulting string=w779:string)  [unwired: 2 in, 1 out]
            }
            frame "Minimum" {
              n249 = Format Into String(format string=":CALC:USER:TRAC6:MARK%d:SEAR:TRAC:TYPE MIN;", w783) -> (resulting string=w782:string)  [unwired: 2 in, 1 out]
            }
            frame "Peak" {
              n250 = Format Into String(format string=":CALC:USER:TRAC6:MARK%d:SEAR:TRAC:TYPE PEAK;", w785) -> (resulting string=w786:string)  [unwired: 2 in, 1 out]
            }
            frame "Target" {
              n251 = Format Into String(format string=":CALC:USER:TRAC6:MARK%d:SEAR:TRAC:TYPE TARG;", w788) -> (resulting string=w789:string)  [unwired: 2 in, 1 out]
            }
            frame "Off", Default {
              n252 = Format Into String(format string=":CALC:USER:TRAC6:MARK%d:SEAR:TRAC:TYPE OFF;", w791) -> (resulting string=w792:string)  [unwired: 2 in, 1 out]
            }
          }
          n253 = case shown="True" w767 {
            tunnel: w763 -> [_ w797]
            tunnel: [":CALC:USER:ALLT:MARK:REF:STAT OFF;" w795] -> w770
            frame False {
            }
            frame True {
              n254 = Format Into String(format string=":CALC:USER:ALLT:MARK:REF:STAT ON;\n:CALC:USER:ALLT:MARK:REF:NUMB %d;", w797) -> (resulting string=w795:string)  [unwired: 2 in, 1 out]
            }
          }
          n255 = case shown="True" w764 {
            tunnel: w763 -> [w774 w777]
            tunnel: [w773 w776] -> w762
            frame False {
              n256 = Format Into String(format string=":CALC:USER:TRAC6:MARK%d:STAT OFF;", w774) -> (resulting string=w773:string)  [unwired: 2 in, 1 out]
            }
            frame True {
              n257 = Format Into String(format string=":CALC:USER:TRAC6:MARK%d:STAT ON;", w777) -> (resulting string=w776:string)  [unwired: 2 in, 1 out]
            }
          }
          n258 = Select(t=":CALC:USER:ALLT:MARK:COUP:STAT ON;", s=w759, f=":CALC:USER:ALLT:MARK:COUP:STAT OFF;") -> (s? t:f=w758:string)
          n259 = Format Into String(format string="%.;:CALC:USER:TRAC6:MARK%d:X %g;", w763, w768) -> (resulting string=w771:string)  [unwired: 2 in, 1 out]
          n260 = Concatenate Strings(w771, w770, w769, w758, w762) -> (w765:string)
        }
        frame 7 {
          # "Trace 7"
          n261 = case shown="\"Off\", Default" w806 {
            tunnel: w804 -> [w821 w823 w825 w828 w831]
            tunnel: [w819 w822 w826 w829 w832] -> w809
            frame "Maximum" {
              n262 = Format Into String(format string=":CALC:USER:TRAC7:MARK%d:SEAR:TRAC:TYPE MAX;", w821) -> (resulting string=w819:string)  [unwired: 2 in, 1 out]
            }
            frame "Minimum" {
              n263 = Format Into String(format string=":CALC:USER:TRAC7:MARK%d:SEAR:TRAC:TYPE MIN;", w823) -> (resulting string=w822:string)  [unwired: 2 in, 1 out]
            }
            frame "Peak" {
              n264 = Format Into String(format string=":CALC:USER:TRAC7:MARK%d:SEAR:TRAC:TYPE PEAK;", w825) -> (resulting string=w826:string)  [unwired: 2 in, 1 out]
            }
            frame "Target" {
              n265 = Format Into String(format string=":CALC:USER:TRAC7:MARK%d:SEAR:TRAC:TYPE TARG;", w828) -> (resulting string=w829:string)  [unwired: 2 in, 1 out]
            }
            frame "Off", Default {
              n266 = Format Into String(format string=":CALC:USER:TRAC7:MARK%d:SEAR:TRAC:TYPE OFF;", w831) -> (resulting string=w832:string)  [unwired: 2 in, 1 out]
            }
          }
          n267 = case shown="True" w807 {
            tunnel: w804 -> [_ w837]
            tunnel: [":CALC:USER:ALLT:MARK:REF:STAT OFF;" w835] -> w810
            frame False {
            }
            frame True {
              n268 = Format Into String(format string=":CALC:USER:ALLT:MARK:REF:STAT ON;\n:CALC:USER:ALLT:MARK:REF:NUMB %d;", w837) -> (resulting string=w835:string)  [unwired: 2 in, 1 out]
            }
          }
          n269 = case shown="True" w803 {
            tunnel: w804 -> [w814 w817]
            tunnel: [w813 w816] -> w802
            frame False {
              n270 = Format Into String(format string=":CALC:USER:TRAC7:MARK%d:STAT OFF;", w814) -> (resulting string=w813:string)  [unwired: 2 in, 1 out]
            }
            frame True {
              n271 = Format Into String(format string=":CALC:USER:TRAC7:MARK%d:STAT ON;", w817) -> (resulting string=w816:string)  [unwired: 2 in, 1 out]
            }
          }
          n272 = Format Into String(format string="%.;:CALC:USER:TRAC7:MARK%d:X %g;", w804, w808) -> (resulting string=w811:string)  [unwired: 2 in, 1 out]
          n273 = Select(t=":CALC:USER:ALLT:MARK:COUP:STAT ON;", s=w799, f=":CALC:USER:ALLT:MARK:COUP:STAT OFF;") -> (s? t:f=w798:string)
          n274 = Concatenate Strings(w811, w810, w809, w798, w802) -> (w805:string)
        }
        frame 8 {
          # "Trace 8"
          n275 = case shown="\"Off\", Default" w846 {
            tunnel: w843 -> [w861 w863 w865 w868 w871]
            tunnel: [w859 w862 w866 w869 w872] -> w849
            frame "Maximum" {
              n276 = Format Into String(format string=":CALC:USER:TRAC8:MARK%d:SEAR:TRAC:TYPE MAX;", w861) -> (resulting string=w859:string)  [unwired: 2 in, 1 out]
            }
            frame "Minimum" {
              n277 = Format Into String(format string=":CALC:USER:TRAC8:MARK%d:SEAR:TRAC:TYPE MIN;", w863) -> (resulting string=w862:string)  [unwired: 2 in, 1 out]
            }
            frame "Peak" {
              n278 = Format Into String(format string=":CALC:USER:TRAC8:MARK%d:SEAR:TRAC:TYPE PEAK;", w865) -> (resulting string=w866:string)  [unwired: 2 in, 1 out]
            }
            frame "Target" {
              n279 = Format Into String(format string=":CALC:USER:TRAC8:MARK%d:SEAR:TRAC:TYPE TARG;", w868) -> (resulting string=w869:string)  [unwired: 2 in, 1 out]
            }
            frame "Off", Default {
              n280 = Format Into String(format string=":CALC:USER:TRAC8:MARK%d:SEAR:TRAC:TYPE OFF;", w871) -> (resulting string=w872:string)  [unwired: 2 in, 1 out]
            }
          }
          n281 = case shown="True" w847 {
            tunnel: w843 -> [_ w877]
            tunnel: [":CALC:USER:ALLT:MARK:REF:STAT OFF;" w875] -> w850
            frame False {
            }
            frame True {
              n282 = Format Into String(format string=":CALC:USER:ALLT:MARK:REF:STAT ON;\n:CALC:USER:ALLT:MARK:REF:NUMB %d;", w877) -> (resulting string=w875:string)  [unwired: 2 in, 1 out]
            }
          }
          n283 = case shown="True" w844 {
            tunnel: w843 -> [w854 w857]
            tunnel: [w853 w856] -> w842
            frame False {
              n284 = Format Into String(format string=":CALC:USER:TRAC8:MARK%d:STAT OFF;", w854) -> (resulting string=w853:string)  [unwired: 2 in, 1 out]
            }
            frame True {
              n285 = Format Into String(format string=":CALC:USER:TRAC8:MARK%d:STAT ON;", w857) -> (resulting string=w856:string)  [unwired: 2 in, 1 out]
            }
          }
          n286 = Format Into String(format string="%.;:CALC:USER:TRAC8:MARK%d:X %g;", w843, w848) -> (resulting string=w851:string)  [unwired: 2 in, 1 out]
          n287 = Select(t=":CALC:USER:ALLT:MARK:COUP:STAT ON;", s=w840, f=":CALC:USER:ALLT:MARK:COUP:STAT OFF;") -> (s? t:f=w839:string)
          n288 = Concatenate Strings(w851, w850, w849, w839, w842) -> (w845:string)
        }
      }
    }
  }
  n289 = VISA Write(VISA resource name="VISA resource name", write buffer=w4, error in (no error)="error in (no error)") -> (VISA resource name out=w8:refnum<visa-resource-name>, error out=w7:errorcluster)  [unwired: 1 out]
  n290 = call "Error Query.vi"("error in (no error)"=w7, "VISA resource name"=w8) -> ("error out"=→"error out":errorcluster, "VISA resource name out"=→"VISA resource name out":refnum<visa-resource-name>)  [unwired: 6 in, 2 out]
